vi "Cliente.vi"() -> ()   [LabVIEW 2021]
panel:
  out "Waveform Chart":dbl(graph)
  in  "Stop":bool
  # "Cliente"
  # "Protocolo:/host/Datos\nPara LabVIEW\ndspt://127.0.0.1/Datos"
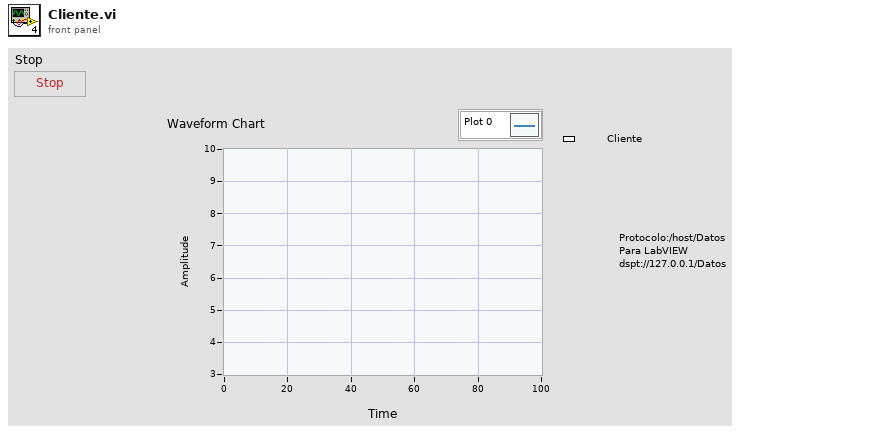
[diagram p1: front panel]
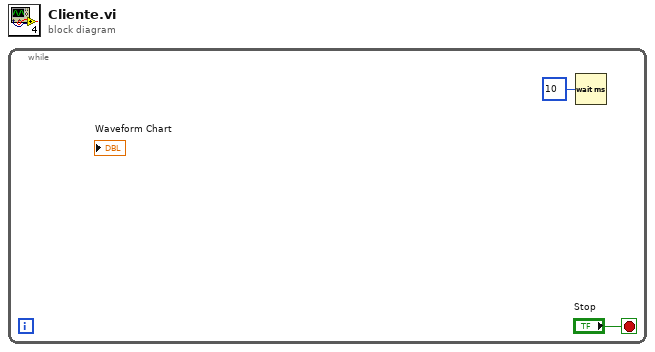
[diagram p0: block diagram]
diagram:
  n1 = while {
    stop <- "Stop" stop-if-true
    n2 = Wait (ms)(milliseconds to wait=u32 10) -> ()  [unwired: 1 out]
  }
